vi "Get Battery Switch States.vi"(8 "error in (no error)":errorcluster, 11 "Item Ref in":T1 format="%.0x") -> (0 "error out":errorcluster, 1 "Battery Switch States":T2[](array[typedef]), 2 "Ordered Battery Switch Channels":T1[](array[typedef]) format="%.0x", 3 "Item Ref out":T1 format="%.0x")   [LabVIEW 2014, in "SLSC configuration System Explorer.lvlib"]
uses:
  SLSC configuration System Explorer.lvlib
  <vilib>/NI Veristand/Custom Device API/Custom Device Item Ref.ctl
  Shared/Battery Switch Board/Battery Switch.ctl
  Shared/Constants.vi
  <vilib>/NI Veristand/Custom Device API/Get Item Property (U16).vi
  <vilib>/NI Veristand/Custom Device API/Custom Device API.lvlib
  Shared/SLSC configuration Shared.lvlib
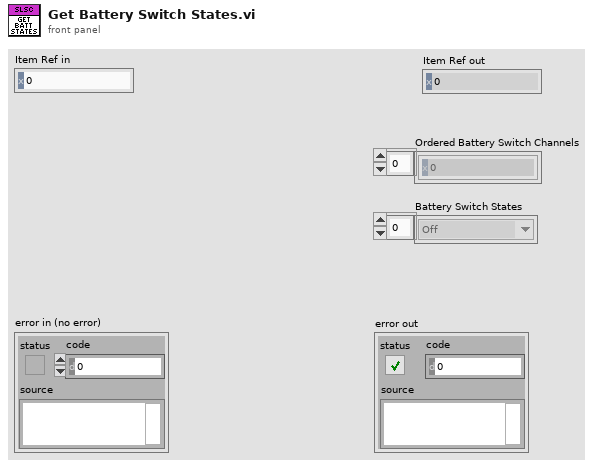
[diagram p1: front panel]
types:
  T1 = typedef "Custom Device API.lvlib/Custom Device Item Ref.ctl" = u64
  T2 = typedef "SLSC configuration Shared.lvlib/Battery Switch.ctl" = enum8{"Off", "On"}
  T3 = typedef "Custom Device API.lvlib/Custom Device Channel.ctl" = cluster{"Type":T4, "Units":string, "Default Value":dbl, "Faultable":bool, "Scalable":bool}
  T4 = typedef "Custom Device API.lvlib/Custom Device Channel Type.ctl" = enum16{"Input", "Output"}
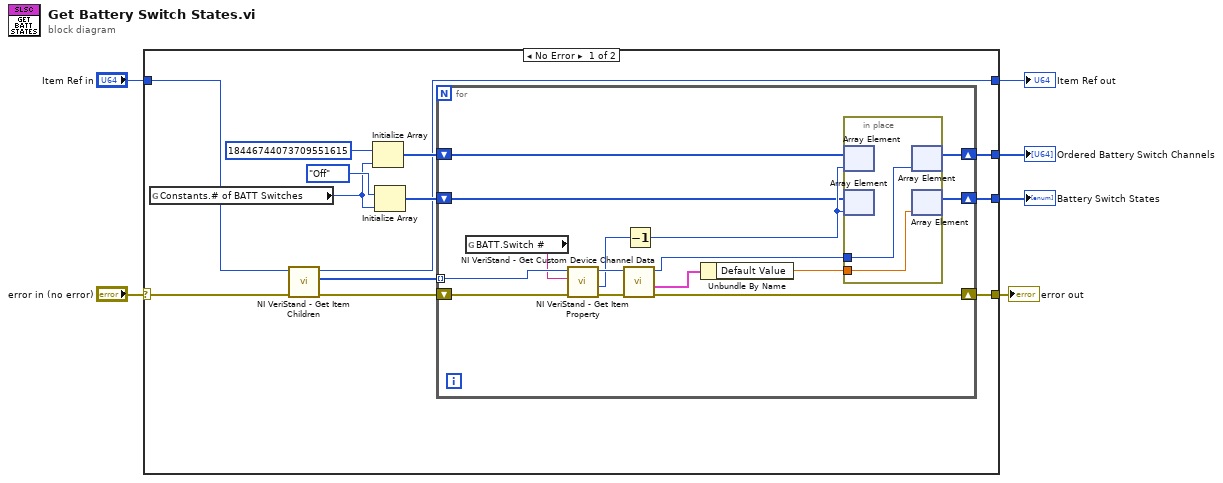
[diagram p0: block diagram]
diagram:
  n1 = case shown="No Error" "error in (no error)" {
    selector: "error in (no error)" -> [w16 w38]
    tunnel: "Item Ref in" -> [w19 w37]
    tunnel: [w10 _] -> w4
    tunnel: [w9 _] -> w3
    tunnel: [w8 w38] -> w2
    tunnel: [w7 w37] -> w1
    frame No Error {
      n2 = global read "Constants.vi" "Constants.# of BATT Switches"() -> (w13:u8)
      n3 = call <vilib>:"NI VeriStand - Get Item Children.vi"("error in (no error)"=w16, "Item Ref in"=w19) -> ("error out"=w17:errorcluster, "Child Refs"=w18:T1[], "Item Ref out"=w7:T1)  [unwired: 6 in, 1 out]
      n4 = Initialize Array(T1 18446744073709551615 ("Item Ref out"), w13) -> (w12:T1[])
      n5 = Initialize Array(Battery_Switch."Off" ("Battery Switch"), w13) -> (w11:T2[])
      n6 = for {
        tunnel: w18 -> [w31] mode=indexing
        shift-right: [w33] -> w8
        shift-left: w17 -> [w32]
        shift-right: [w21] -> w9
        shift-left: w11 -> [w24]
        shift-right: [w20] -> w10
        shift-left: w12 -> [w25]
        n7 = global read "Constants.vi" "BATT.Switch #"() -> (w30:string)
        n8 = call-poly <vilib>:"NI VeriStand - Get Item Property.vi"("error in (no error)"=w32, "Property Name"=w30, "Item Ref in"=w31) -> ("error out"=w29:errorcluster, "Value"=w27:u16, "Item Ref out"=w28:T1)  [unwired: 5 in, 1 out]
        n9 = call <vilib>:"NI VeriStand - Get Custom Device Channel Data.vi"("error in (no error)"=w29, "Channel Ref in"=w28) -> ("error out"=w33:errorcluster, "Channel"=w34:T3, "Channel Ref out"=w22:T1)  [unwired: 4 in, 3 out]
        n10 = Decrement(x=w27) -> (x-1=w26:u16)
        n11 = Unbundle By Name(w34) -> ("Default Value"=w23:dbl)
        n12 = in-place {
          in-place-border: w23 -> [w36]
          in-place-border: w22 -> [w35]
          n13 = in-place-array #1(w25, w26) -> ()  [unwired: 1 out]
          n14 = in-place-array #2(w24, w26) -> ()  [unwired: 1 out]
          n15 = in-place-array #1(w35) -> (w20:T1[])  [unwired: 1 out]
          n16 = in-place-array #2(w36) -> (w21:T2[])  [unwired: 1 out]
        }
      }
    }
    frame Error {
    }
  }
  "Ordered Battery Switch Channels" <- w4
  "Battery Switch States" <- w3
  "error out" <- w2
  "Item Ref out" <- w1
